vi "RxPkt - Add Packet.vi"(8 "error in (no error)":errorcluster, 9 "New Packet ID":i32, 10 "New Packet Name":string, 11 "Item Ref in":T1=18446744073709551615 format="%.0x") -> (0 "error out":errorcluster, 2 "New Packet Ref":T1=18446744073709551615 format="%.0x", 3 "Item Ref Out":T1=18446744073709551615 format="%.0x")   [LabVIEW 2016, in "UDP-Custom-Device System Explorer.lvlib"]
uses:
  UDP-Custom-Device System Explorer.lvlib
  <vilib>/NI Veristand/Custom Device API/Custom Device Item Ref.ctl
  <vilib>/NI Veristand/Custom Device API/Custom Device Channel.ctl
  <vilib>/NI Veristand/Custom Device API/Custom Device Channel Type.ctl
  Shared/Constants.vi
  Shared/UDP-Custom-Device Shared.lvlib
  <vilib>/NI VeriStand/Custom Device API/Custom Device API.lvlib
  Property Accessors/Shared Section Accessors.lvlib
  Property Accessors/Shared Packet Accessors.lvlib
panel:
  out "error out 3":errorcluster
  out "error out 2":errorcluster
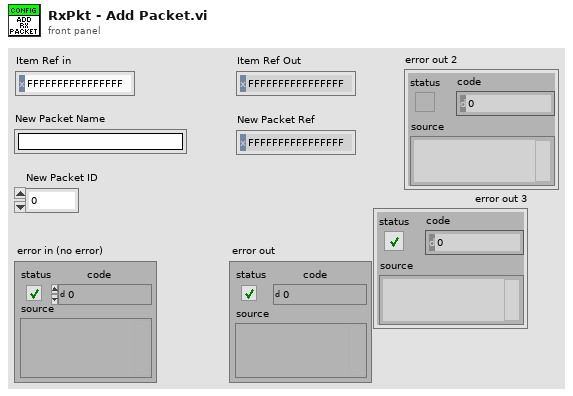
[diagram p1: front panel]
types:
  T1 = typedef "Custom Device API.lvlib/Custom Device Item Ref.ctl" = u64
  T2 = typedef "Custom Device API.lvlib/Custom Device Channel.ctl" = cluster{"Type":T3, "Units":string, "Default Value":dbl, "Faultable":bool, "Scalable":bool}
  T3 = typedef "Custom Device API.lvlib/Custom Device Channel Type.ctl" = enum16{"Input", "Output"}
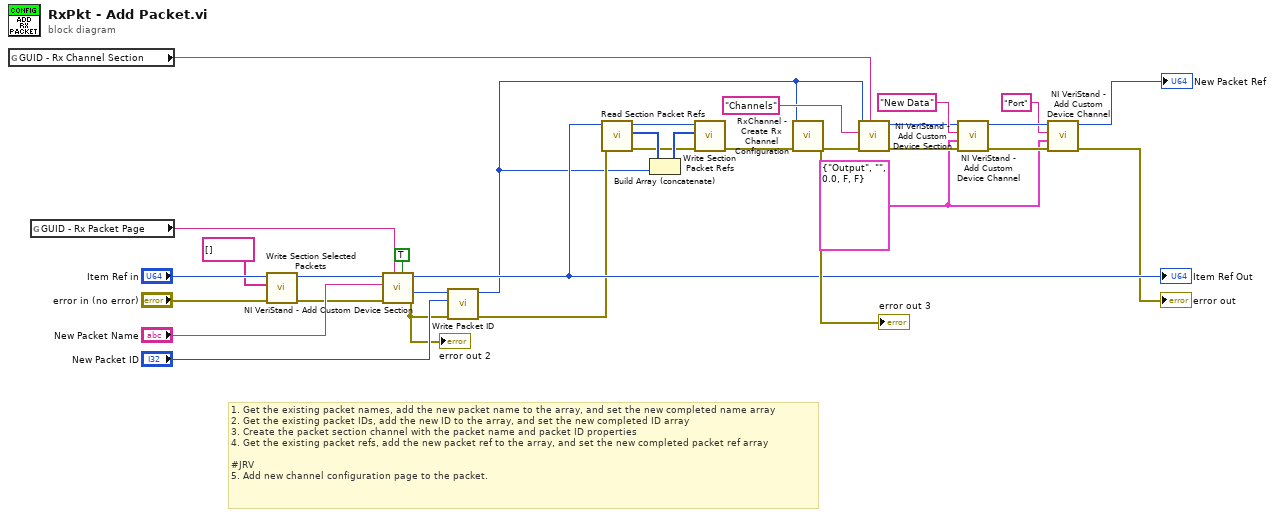
[diagram p0: block diagram]
diagram:
  w1 = T2 {"Type"=enum."Output", "Units"="", "Default Value"=0.0, "Faultable"=FALSE, "Scalable"=FALSE} ("Channel")
  # "1. Get the existing packet names, add the new packet name to the array, and set the new completed name array\n2. Get the existing packet IDs, add the new ID to the array, and set the new completed ID array\n3. Create the packet section channel with the packet name and packet ID properties\n4. Get the existing packet refs, add the new packet ref to the array, and set the new completed packet ref array\n\n#JRV\n5. Add new channel configuration page to the packet."
  n1 = global read "Constants.vi" "GUID - Rx Channel Section"() -> (w26:string)
  n2 = global read "Constants.vi" "GUID - Rx Packet Page"() -> (w30:string)
  n3 = call "Write Section Selected Packets.vi"("error in (no error)"="error in (no error)", "Selected Packets"=string[] [] ("Value"), "Node Ptr"="Item Ref in") -> ("error out"=w16:errorcluster, "Node Ptr out"=w18:T1)  [unwired: 7 in]
  n4 = call <vilib>:"NI VeriStand - Add Custom Device Section.vi"("Highlight? (F)"=TRUE, "GUID (Default Section)"=w30, "error in (no error)"=w16, "Section Name"="New Packet Name", "Parent Ref in"=w18) -> ("error out"=w12:errorcluster, "Section Ptr"=w13:T1, "Parent Ref out"=w25:T1)  [unwired: 3 in, 1 out]
  "Item Ref Out" <- w25
  "error out 2" <- w12
  n5 = call "Write Packet ID.vi"("error in (no error)"=w12, "Packet ID"="New Packet ID", "Node Ptr"=w13) -> ("error out"=w11:errorcluster, "Node Ptr out"=w8:T1)  [unwired: 7 in]
  n6 = call "Read Section Packet Refs.vi"("error in (no error)"=w11, "Node Ptr"=w25) -> ("error out"=w21:errorcluster, "Dependent Node Refs"=w24:T1[], "Node Ptr out"=w23:T1)  [unwired: 7 in]
  n7 = Build Array (concatenate)(w24, w8) -> (w22:T1[])
  n8 = call "Write Section Packet Refs.vi"("error in (no error)"=w21, "Dependent Node Refs"=w22, "Node Ptr"=w23) -> ("error out"=w20:errorcluster)  [unwired: 7 in, 1 out]
  n9 = call "RxChannel - Create Rx Channel Configuration.vi"("error in (no error)"=w20, "Parent Packet Ref"=w8) -> ("error out"=w27:errorcluster)  [unwired: 8 in, 1 out]
  "error out 3" <- w27
  n10 = call <vilib>:"NI VeriStand - Add Custom Device Section.vi"("GUID (Default Section)"=w26, "error in (no error)"=w27, "Section Name"="Channels", "Parent Ref in"=w8) -> ("error out"=w7:errorcluster, "Parent Ref out"=w9:T1)  [unwired: 4 in, 2 out]
  n11 = call <vilib>:"NI VeriStand - Add Custom Device Channel.vi"("error in (no error)"=w7, "Channel"=w1, "Channel Name"="New Data", "Parent Ref in"=w9) -> ("error out"=w4:errorcluster, "Parent Ref out"=w6:T1)  [unwired: 4 in, 2 out]
  n12 = call <vilib>:"NI VeriStand - Add Custom Device Channel.vi"("error in (no error)"=w4, "Channel"=w1, "Channel Name"="Port", "Parent Ref in"=w6) -> ("error out"=→"error out":errorcluster, "Parent Ref out"=→"New Packet Ref":T1)  [unwired: 4 in, 2 out]
